vi "ATT Driver Test.vi"() -> ()   [LabVIEW 2011]
uses:
  SWI/SWI Command.ctl
  SWI/SWI Driver Ref.ctl
panel:
  in  "write-read":bool
  in  "read":bool
  in  "write":bool
  in  "preset":bool
  in  "config":bool
  in  "init":bool
  in  "SWI Drivers":u16(ring) items=["Sea-Level SWI"]
  in  "load":bool
  in  "stop":bool
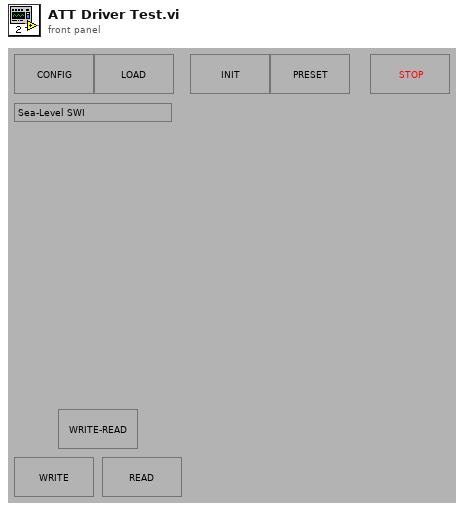
[diagram p1: front panel]
types:
  T1 = typedef "SWI Driver Ref.ctl" = refnum<vi>
  T2 = typedef "SWI Command.ctl" = enum16{"LOAD", "INITIALIZE", "PRESET", "SET STIMULUS", "GET STIMULUS", "GET INFO", "RELEASE", "UNLOAD"}
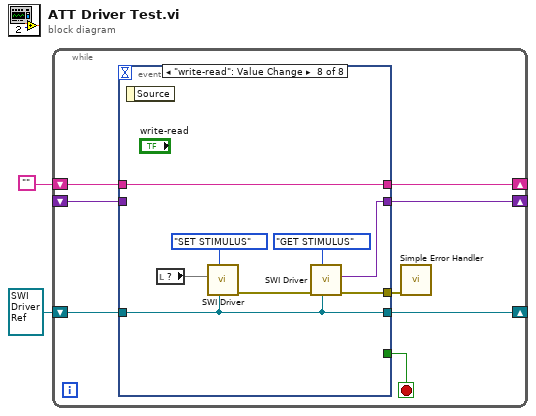
[diagram p0: block diagram]
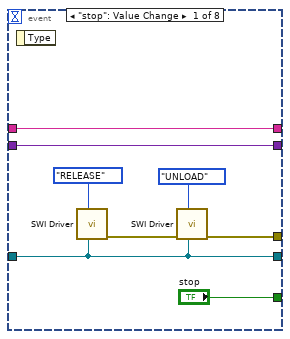
[diagram p2: hidden frame]
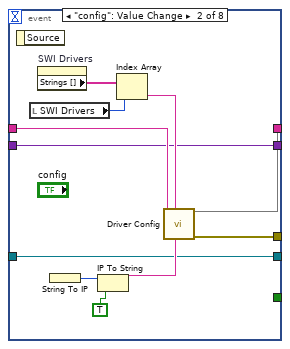
[diagram p3: hidden frame]
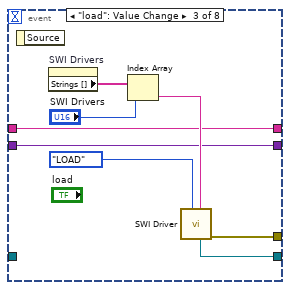
[diagram p4: hidden frame]
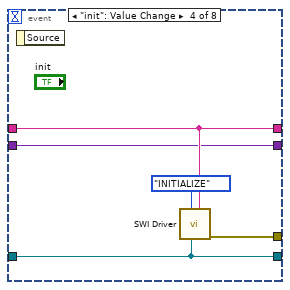
[diagram p5: hidden frame]
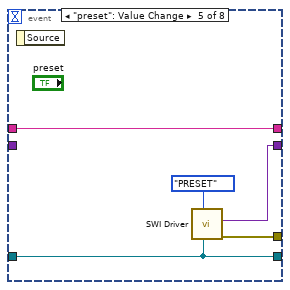
[diagram p6: hidden frame]
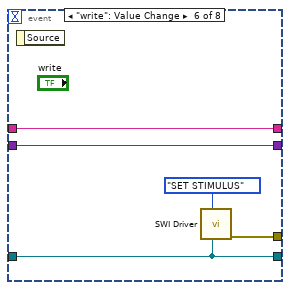
[diagram p7: hidden frame]
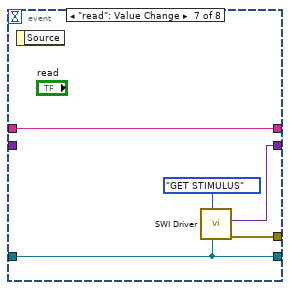
[diagram p8: hidden frame]
diagram:
  n1 = while {
    shift-right: [w8] -> _
    shift-left: "" -> [w7]
    shift-right: [w5] -> _
    shift-left: T1 refnum ("Driver Ref") -> [w6]
    shift-right: [w3] -> _
    shift-left: _ -> [w4]
    stop <- w10 stop-if-true
    n2 = event shown="[7] \"write-read\": Value Change" {
      selector: _ -> [_ _ _ _ _ _ _ _]
      dyn-events: _ -> [_ _ _ _ _ _ _ _]
      timeout: _ -> [_ _ _ _ _ _ _ _]
      tunnel: ["stop" _ _ _ _ _ _ _] -> w10
      tunnel: [w14 w29 w33 w42 w47 w51 w56 w64] -> w9
      tunnel: [w17 w28 w32 w39 w46 w53 w58 w66] -> w8
      tunnel: w7 -> [w17 w27 w32 w39 w46 w53 w58 w66]
      tunnel: w6 -> [w12 w20 _ w40 w44 w50 w55 w60]
      tunnel: [w12 w20 w31 w40 w44 w50 w55 w60] -> w5
      tunnel: [w11 w19 w30 w38 w43 w48 w54 w63] -> w3
      tunnel: w4 -> [w11 w19 w30 w38 _ w48 _ _]
      event "stop": Value Change {
        n3 = event-data() -> ()  [unwired: 1 in, 1 out]
        n4 = call "SWI Driver.vi"("Drv Refnum"=w12, "SWI Command"=SWI_Command."RELEASE" ("VNA Command")) -> ("error out"=w15:errorcluster)  [unwired: 6 in, 3 out]
        n5 = call "SWI Driver.vi"("Drv Refnum"=w12, "SWI Command"=SWI_Command."UNLOAD" ("VNA Command"), "error in (no error)"=w15) -> ("error out"=w14:errorcluster)  [unwired: 5 in, 3 out]
      }
      event "config": Value Change {
        n6 = event-data() -> ()  [unwired: 1 in, 1 out]
        n7 = local read "SWI Drivers"() -> (w23:u16)
        n8 = property on="SWI Drivers" class="Ring (strict)"() -> ("Strings []"=w22:string[])  [unwired: 2 in, 2 out]
        n9 = String To IP() -> (0:w26:u32)  [unwired: 1 in]
        n10 = IP To String(1:TRUE, 2:w26) -> (0:w25:string)
        n11 = Index Array(array=w22, index=w23) -> (element=w21:string)
        n12 = call "Driver Config.vi"("CalDue"=w25, "DriverType (\"\")"=w21, "TestStation Client (\"\")"=w27) -> ("error out"=w29:errorcluster, 3:w28)  [unwired: 4 in, 3 out]
      }
      event "load": Value Change {
        n13 = event-data() -> ()  [unwired: 1 in, 1 out]
        n14 = property on="SWI Drivers" class="Ring (strict)"() -> ("Strings []"=w36:string[])  [unwired: 2 in, 2 out]
        n15 = Index Array(array=w36, index="SWI Drivers") -> (element=w34:string)
        n16 = call "SWI Driver.vi"("SWI Configuration (\"\")"=w34, "SWI Command"=SWI_Command."LOAD" ("VNA Command")) -> ("error out"=w33:errorcluster, "dup Drv Refnum"=w31:T1)  [unwired: 6 in, 2 out]
      }
      event "init": Value Change {
        n17 = event-data() -> ()  [unwired: 1 in, 1 out]
        n18 = call "SWI Driver.vi"("SWI Configuration (\"\")"=w39, "Drv Refnum"=w40, "SWI Command"=SWI_Command."INITIALIZE" ("VNA Command")) -> ("error out"=w42:errorcluster)  [unwired: 5 in, 3 out]
      }
      event "preset": Value Change {
        n19 = event-data() -> ()  [unwired: 1 in, 1 out]
        n20 = call "SWI Driver.vi"("Drv Refnum"=w44, "SWI Command"=SWI_Command."PRESET" ("VNA Command")) -> ("error out"=w47:errorcluster, "SWI Position Out"=w43:variant)  [unwired: 6 in, 2 out]
      }
      event "write": Value Change {
        n21 = event-data() -> ()  [unwired: 1 in, 1 out]
        n22 = call "SWI Driver.vi"("Drv Refnum"=w50, "SWI Command"=SWI_Command."SET STIMULUS" ("VNA Command")) -> ("error out"=w51:errorcluster, "SWI Position In"=w49:variant)  [unwired: 5 in, 3 out]
      }
      event "read": Value Change {
        n23 = event-data() -> ()  [unwired: 1 in, 1 out]
        n24 = call "SWI Driver.vi"("Drv Refnum"=w55, "SWI Command"=SWI_Command."GET STIMULUS" ("VNA Command")) -> ("error out"=w56:errorcluster, "SWI Position Out"=w54:variant)  [unwired: 6 in, 2 out]
      }
      event "write-read": Value Change {
        n25 = event-data() -> ()  [unwired: 1 in, 1 out]
        n26 = local read item#-1() -> (w59)
        n27 = call "SWI Driver.vi"("Drv Refnum"=w60, "SWI Command"=SWI_Command."SET STIMULUS" ("VNA Command"), "SWI Position In"=w59) -> ("error out"=w61:errorcluster)  [unwired: 5 in, 3 out]
        n28 = call "SWI Driver.vi"("Drv Refnum"=w60, "SWI Command"=SWI_Command."GET STIMULUS" ("VNA Command"), "error in (no error)"=w61) -> ("error out"=w64:errorcluster, "SWI Position Out"=w63:variant)  [unwired: 5 in, 2 out]
      }
    }
    n29 = call <vilib>:"Simple Error Handler.vi"("error in (no error)"=w9) -> ()  [unwired: 4 in, 5 out]
  }
